vi "WireWriteTagbusVIs.vi"(5 "terminals data":refnum<vi>[](array[refnum]), 7 "terminals indexes":refnum<vi>[](array[refnum]), 8 "error in":errorcluster, 9 "elements in cluster":i32, 10 "tag bus in in":refnum<vi>, 11 "VI in":refnum<vi>) -> (0 "error out":errorcluster, 2 "tag bus out":refnum<vi>, 3 "VI out":refnum<vi>)   [LabVIEW 2013]
uses:
  <vilib>/Utility/miscctls.llb/LVPointTypeDef.ctl
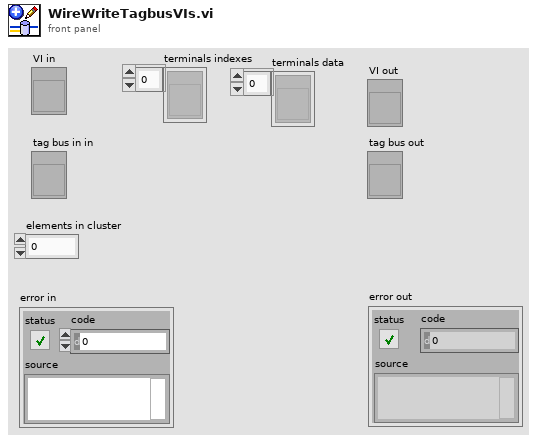
[diagram p1: front panel]
types:
  T1 = typedef "LVPointTypeDef.ctl" = cluster{"Horizontal":i16, "Vertical":i16}
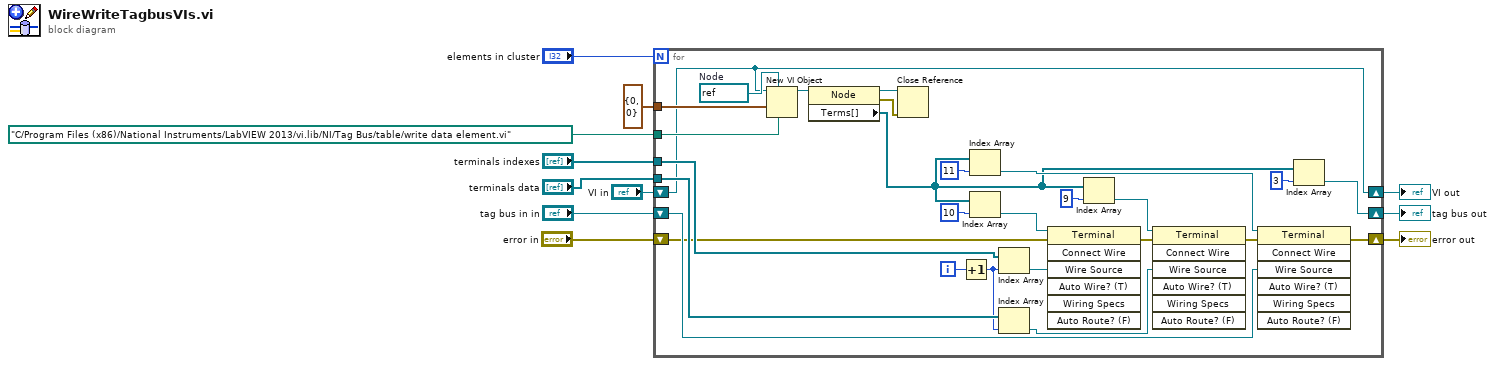
[diagram p0: block diagram]
diagram:
  n1 = for {
    N: "elements in cluster" -> [_]
    tunnel: path "C:/Program Files (x86)/National Instruments/LabVIEW 2013/vi.lib/NI/Tag Bus/table/write data element.vi" ("path") -> [w38]
    tunnel: T1 {"Horizontal"=0, "Vertical"=0} ("location") -> [w37]
    tunnel: "terminals data" -> [w29]
    tunnel: "terminals indexes" -> [w26]
    shift-right: [w20] -> w9
    shift-left: "tag bus in in" -> [w23]
    shift-right: [w17] -> w8
    shift-left: "VI in" -> [w17]
    shift-right: [w12] -> w1
    shift-left: "error in" -> [w13]
    i -> [w19]
    w36 = refnum<vi> refnum  # Node
    n2 = New VI Object(vi object class=w36, owner refnum=w17, position/next to=w37, 6:w38) -> (object refnum=w31:refnum<vi>)  [unwired: 4 in, 1 out]
    n3 = property on="Property Node" class="Node"(reference=w31) -> (reference out=w33:refnum<vi>, error out=w32:errorcluster, "Terms[]"=w16:refnum<vi>[])  [unwired: 1 in]
    n4 = Close Reference(reference=w33, error in (no error)=w32) -> ()  [unwired: 1 out]
    n5 = Increment(x=w19) -> (x+1=w18:i32)
    n6 = Index Array(array=w16, index=11) -> (element=w22:refnum<vi>)
    n7 = Index Array(array=w16, index=10) -> (element=w27:refnum<vi>)
    n8 = Index Array(array=w26, index=w18) -> (element=w25:refnum<vi>)
    n9 = Index Array(array=w29, index=w18) -> (element=w28:refnum<vi>)
    n10 = invoke on="Invoke Node" class="Terminal" method="Connect Wire"(reference=w27, error in=w13, "Wire Source"=w25) -> (error out=w15:errorcluster)  [unwired: 4 in, 6 out]
    n11 = Index Array(array=w16, index=9) -> (element=w30:refnum<vi>)
    n12 = invoke on="Invoke Node" class="Terminal" method="Connect Wire"(reference=w30, error in=w15, "Wire Source"=w28) -> (error out=w14:errorcluster)  [unwired: 4 in, 6 out]
    n13 = invoke on="Invoke Node" class="Terminal" method="Connect Wire"(reference=w22, error in=w14, "Wire Source"=w23) -> (error out=w12:errorcluster)  [unwired: 4 in, 6 out]
    n14 = Index Array(array=w16, index=3) -> (element=w20:refnum<vi>)
  }
  "tag bus out" <- w9
  "VI out" <- w8
  "error out" <- w1
